vi "NYStylePepperoniPizza.vi"(8 "error in (no error)":errorcluster) -> (0 "error out":errorcluster, 3 "NYStylePepperoniPizza":refnum<class "NYStylePepperoniPizza.lvclass">)   [LabVIEW 2020, in "FactoryMethod.lvlib" / "PizzaFactoryMethod.lvlib" / "NYStylePepperoniPizza.lvclass"]
uses:
  NYStylePepperoniPizza.lvclass
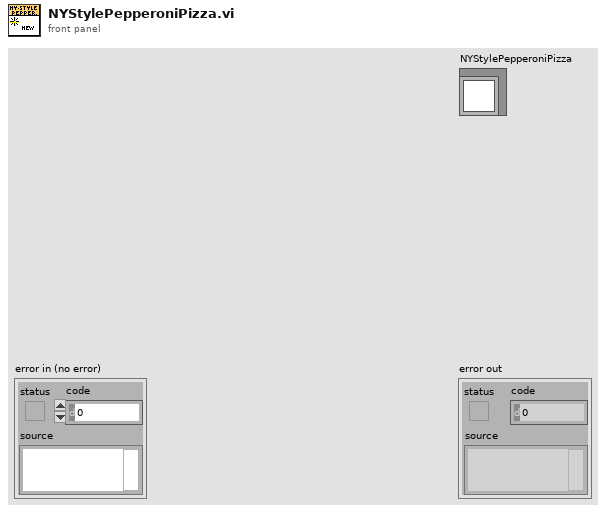
[diagram p1: front panel]
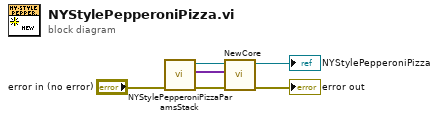
[diagram p0: block diagram]
diagram:
  n1 = call "NYStylePepperoniPizzaParamsStack.vi"("error iN"="error in (no error)") -> ("error out"=w6:errorcluster, "HierarchyParams"=w5:variant[], "NYStylePepperoniPizza"=w1:refnum<class "NYStylePepperoniPizza.lvclass">)  [unwired: 8 in]
  n2 = call-dynamic "NewCore.vi"("error in (no error)"=w6, "ParamsArray"=w5, "NYStylePepperoniPizza"=w1) -> ("error out"=→"error out":errorcluster, "NYStylePepperoniPizza"=→"NYStylePepperoniPizza":refnum<class "NYStylePepperoniPizza.lvclass">)  [unwired: 7 in]
